vi "Get TC Reference.vi"(8 "error in (no error)":errorcluster, 11 "VISA resource name":refnum<visa-resource-name>) -> (0 "error out":errorcluster, 1 "External Reference Value":dbl format="%.4f", 2 "Reference Source":u16, 3 "VISA resource name out":refnum<visa-resource-name>, 4 "Temperature Units":i32)   [LabVIEW 2014, in "Fluke 5XXX Series Multicalibrators.lvlib"]
doc: "This VI returns the source and value of the temperature being used as a reference for thermocouple simulation and measurement (in Celsius, CEL, or Fahrenheit, FAR, depending on active units).\n\nNote:\n\nThis VI is available only for instrument models 5500A and 5520A."
uses:
  Fluke 5XXX Series Multicalibrators.lvlib
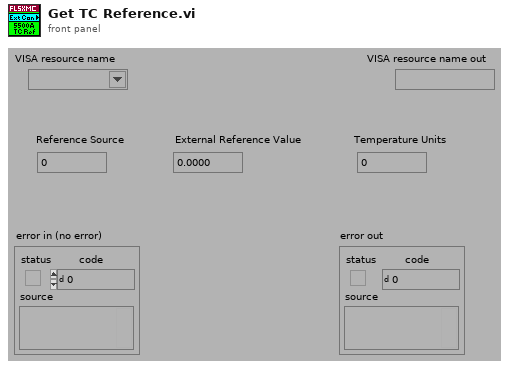
[diagram p1: front panel]
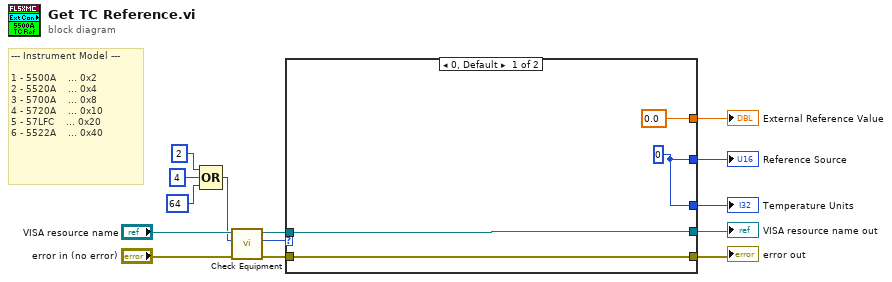
[diagram p0: block diagram]
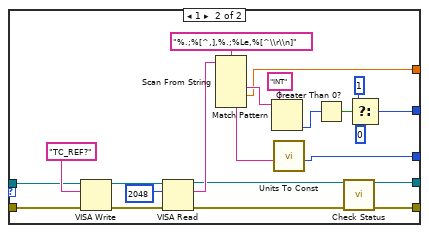
[diagram p2: hidden frame]
diagram:
  # "--- Instrument Model ---\n\n1 - 5500A    ... 0x2\n2 - 5520A    ... 0x4\n3 - 5700A    ... 0x8\n4 - 5720A    ... 0x10\n5 - 57LFC    ... 0x20\n6 - 5522A    ... 0x40"
  n1 = Compound Arithmetic op=OR(2 ("Numeric"), 4 ("Numeric"), 64 ("Numeric")) -> (w1:i32)
  n2 = call "Check Equipment.vi"("error in (no error)"="error in (no error)", "Bit Mask"=w1, "VISA resource name"="VISA resource name") -> ("error out"=w14:errorcluster, "Present?"=w13:u32, "VISA resource name out"=w12:refnum<visa-resource-name>)  [unwired: 6 in]
  n3 = case shown="0, Default" w13 {
    tunnel: [w18 w34] -> w9
    tunnel: [w17 w33] -> w8
    tunnel: w14 -> [w18 w36]
    tunnel: w12 -> [w17 w35]
    tunnel: [w15 w24] -> w7
    tunnel: [0.0 w23] -> w6
    tunnel: [w15 w22] -> w5
    frame 0, Default {
      w15 = u16 0
    }
    frame 1 {
      n4 = VISA Write(VISA resource name=w35, write buffer="TC_REF?", error in (no error)=w36) -> (VISA resource name out=w39:refnum<visa-resource-name>, error out=w38:errorcluster)  [unwired: 1 out]
      n5 = VISA Read(VISA resource name=w39, byte count=u32 2048 ("byte count (0)"), error in (no error)=w38) -> (VISA resource name out=w20:refnum<visa-resource-name>, read buffer=w26:string, error out=w21:errorcluster)  [unwired: 1 out]
      n6 = Scan From String(format string="%.;%[^,],%.;%Le,%[^\\r\\n]", input string=w26) -> (output 1=w25:string, output 2=w23:dbl, output 3=w19:string)  [unwired: 5 in, 3 out]
      n7 = Match Pattern(string=w25, regular expression="INT") -> (offset past match=w30:i32)  [unwired: 1 in, 3 out]
      n8 = call "Units To Const.vi"("Units"=w19) -> ("Const"=w22:i32)  [unwired: 10 in]
      n9 = Greater Than 0?(x=w30) -> (x > 0?=w27:bool)
      n10 = call "Check Status.vi"("VISA resource name"=w20, "error in (no error)"=w21) -> ("VISA resource name out"=w33:refnum<visa-resource-name>, "error out"=w34:errorcluster)  [unwired: 12 in]
      n11 = Select(t=u16 1 ("f"), s=w27, f=u16 0) -> (s? t:f=w24:u16)
    }
  }
  "Reference Source" <- w7
  "External Reference Value" <- w6
  "Temperature Units" <- w5
  "VISA resource name out" <- w8
  "error out" <- w9
